vi "Get Parameter Definition.vi"(8 "error in":errorcluster, 11 "parameter ref in":T1 format="%.0x") -> (0 "error out":errorcluster, 2 "parameter definition":T2, 3 "parameter ref out":T1 format="%.0x")   [LabVIEW 2020, in "ARINC 429 Scripting.lvlib"]
uses:
  ARINC 429 Scripting.lvlib
  Shared/Parameter Definition.ctl
  Encoding and Decoding/Encoding.ctl
  <vilib>/NI VeriStand/Custom Device API/Custom Device Item Ref.ctl
  Encoding and Decoding/Encoding and Decoding.lvlib
  <vilib>/NI VeriStand/Custom Device API/Custom Device API.lvlib
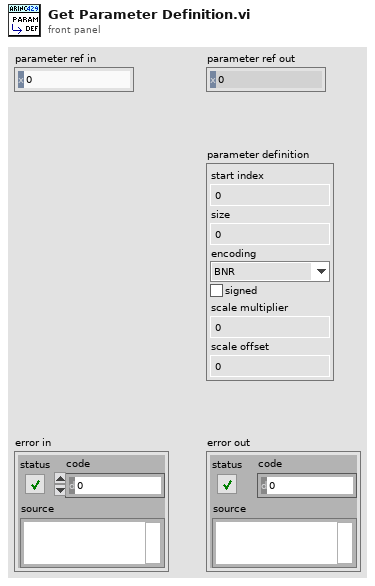
[diagram p1: front panel]
types:
  T1 = typedef "Custom Device API.lvlib/Custom Device Item Ref.ctl" = u64
  T2 = typedef "Parameter Definition.ctl" = cluster{"start index":i32, "size":i32, "encoding":T3, "signed":bool, "scale multiplier":dbl, "scale offset":dbl}
  T3 = typedef "Encoding and Decoding.lvlib/Encoding.ctl" = enum16{"BNR", "BCD", "Discrete"}
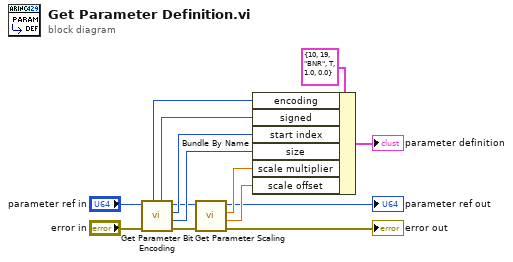
[diagram p0: block diagram]
diagram:
  n1 = call "Get Parameter Bit Encoding.vi"("error in"="error in", "parameter ref in"="parameter ref in") -> ("error out"=w4:errorcluster, "number of bits"=w11:i32, "start bit"=w10:i32, "parameter ref out"=w3:T1, "signed?"=w9:bool, "encoding type"=w8:T3)  [unwired: 4 in]
  n2 = call "Get Parameter Scaling.vi"("error in (no error)"=w4, "parameter ref in"=w3) -> ("error out"=→"error out":errorcluster, "scale offset"=w13:dbl, "scale multiplier"=w12:dbl, "parameter ref out"=→"parameter ref out":T1)  [unwired: 6 in]
  n3 = Bundle By Name(cluster=T2 {"start index"=10, "size"=19, "encoding"=enum."BNR", "signed"=TRUE, "scale multiplier"=1.0, "scale offset"=0.0} ("parameter definition in"), "encoding"=w8, "signed"=w9, "start index"=w10, "size"=w11, "scale multiplier"=w12, "scale offset"=w13) -> (→"parameter definition":T2)
